vi "Set Strings from Ref.vi"(8 "error in (no error)":errorcluster, 9 "Language Index (0)":i32, 10 "GObj Refnum":refnum<vi>, 11 "BoolControl in":refnum<class "BoolControl.lvclass">) -> (0 "error out":errorcluster, 3 "BoolControl out":refnum<class "BoolControl.lvclass">)   [LabVIEW 2013, in "SET Project Data.lvlib" / "BoolControl.lvclass"]
uses:
  BoolControl.lvclass
  Control/Control.lvclass
  SET Project Data.lvlib
  GObject/GObject.lvclass
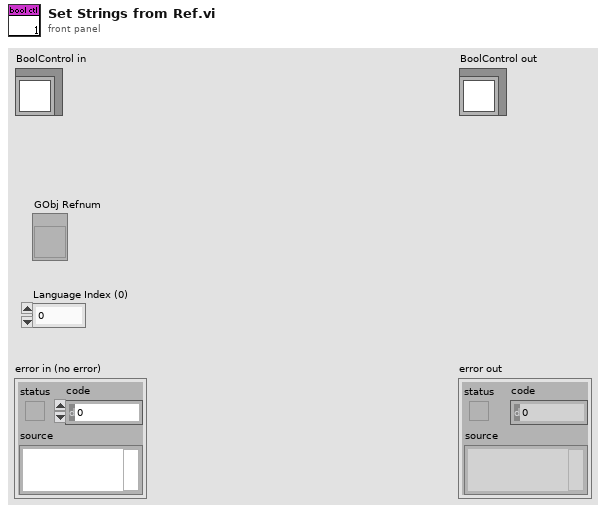
[diagram p1: front panel]
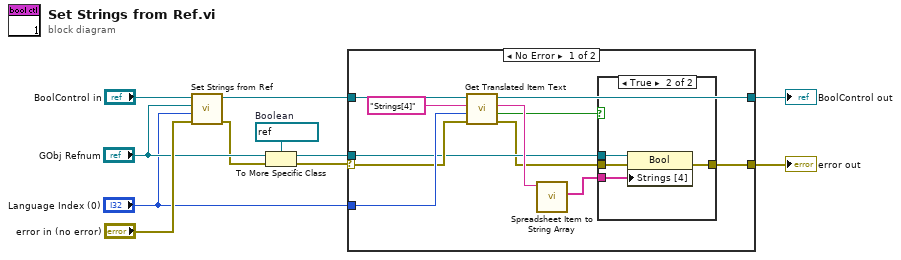
[diagram p0: block diagram]
diagram:
  w8 = refnum<vi> refnum  # Boolean
  n1 = call-parent "Set Strings from Ref.vi"("error in (no error)"="error in (no error)", "Language Index (0)"="Language Index (0)", "GObj Refnum"="GObj Refnum", "Control in"="BoolControl in") -> ("error out"=w7:errorcluster, "Control out"=w4:refnum<class "BoolControl.lvclass">)  [unwired: 6 in]
  n2 = To More Specific Class(target class=w8, reference="GObj Refnum", error in=w7) -> (specific class reference=w5:refnum<vi>, error out=w6:errorcluster)
  n3 = case shown="No Error" w6 {
    selector: w6 -> [w17 w28]
    tunnel: w5 -> [w15 _]
    tunnel: w4 -> [w21 w29]
    tunnel: "Language Index (0)" -> [w20 _]
    tunnel: [w19 w29] -> w2
    tunnel: [w12 w28] -> w1
    frame No Error {
      n4 = call "Get Translated Item Text.vi"("error in (no error)"=w17, "LangIndex (0)"=w20, "ItemName"="Strings[4]", "GObject in"=w21) -> ("error out"=w13:errorcluster, "Found?"=w16:bool, "Translated Text (ASCII)"=w18:string, "GObject out"=w19:refnum<class "BoolControl.lvclass">)  [unwired: 4 in]
      n5 = call "Spreadsheet Item to String Array.vi"("Spreadsheet Item (ASCII)"=w18) -> ("Strings [] (ASCII)"=w14:string[])  [unwired: 10 in]
      n6 = case shown="True" w16 {
        tunnel: w15 -> [_ w27]
        tunnel: w14 -> [_ w26]
        tunnel: w13 -> [w23 w25]
        tunnel: [w23 w24] -> w12
        frame False {
        }
        frame True {
          n7 = property class="Bool"(reference=w27, error in=w25, "Strings [4]"=w26) -> (error out=w24:errorcluster)  [unwired: 1 out]
        }
      }
    }
    frame Error {
    }
  }
  "error out" <- w1
  "BoolControl out" <- w2
